vi "Simple Network Streams - Target.vi"() -> ()   [LabVIEW 2023]
doc: "Demonstrates how to use Network Streams to pass data and commands between two running VIs. This VI passes data to the host VI, based on the frequency specified by the host VI."
uses:
  support/Network Stream Command.ctl
  support/Network Stream Global Stop.vi
  <vilib>/ErrorRing/Error Ring.xnode
  <resource>/objmgr/ni.dex.rc
panel:
  out "Write Backlog":i32
  in  "Write Speed":u16(ring)=1 items=["Fast (10 ms)", "Slow (20 ms)"]
  out "Frequency":dbl(knob) scale=10.0..100.0
  in  "Stop":bool
  # "Overview: Demonstrates how to use Network Streams to pass data and commands between two running VIs.\nRequirements: Windows\nInstructions:\n1. Run this VI.\n2. Open Simple Network Streams - Host.vi and follow the instructions on its front panel."
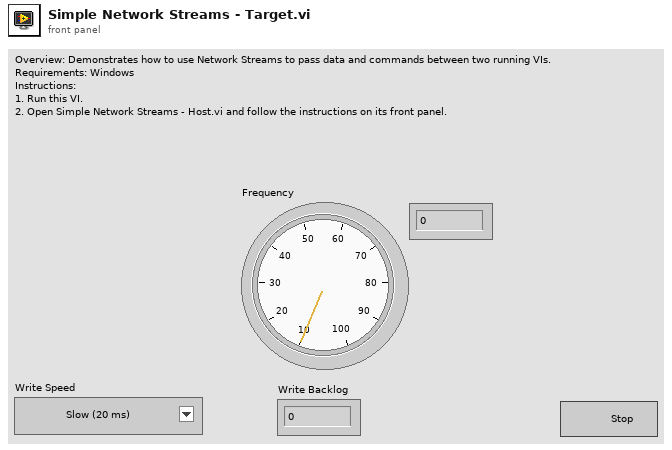
[diagram p1: front panel]
types:
  T1 = typedef "Network Stream Command.ctl" = cluster{"Message":string, "Message Data":variant}
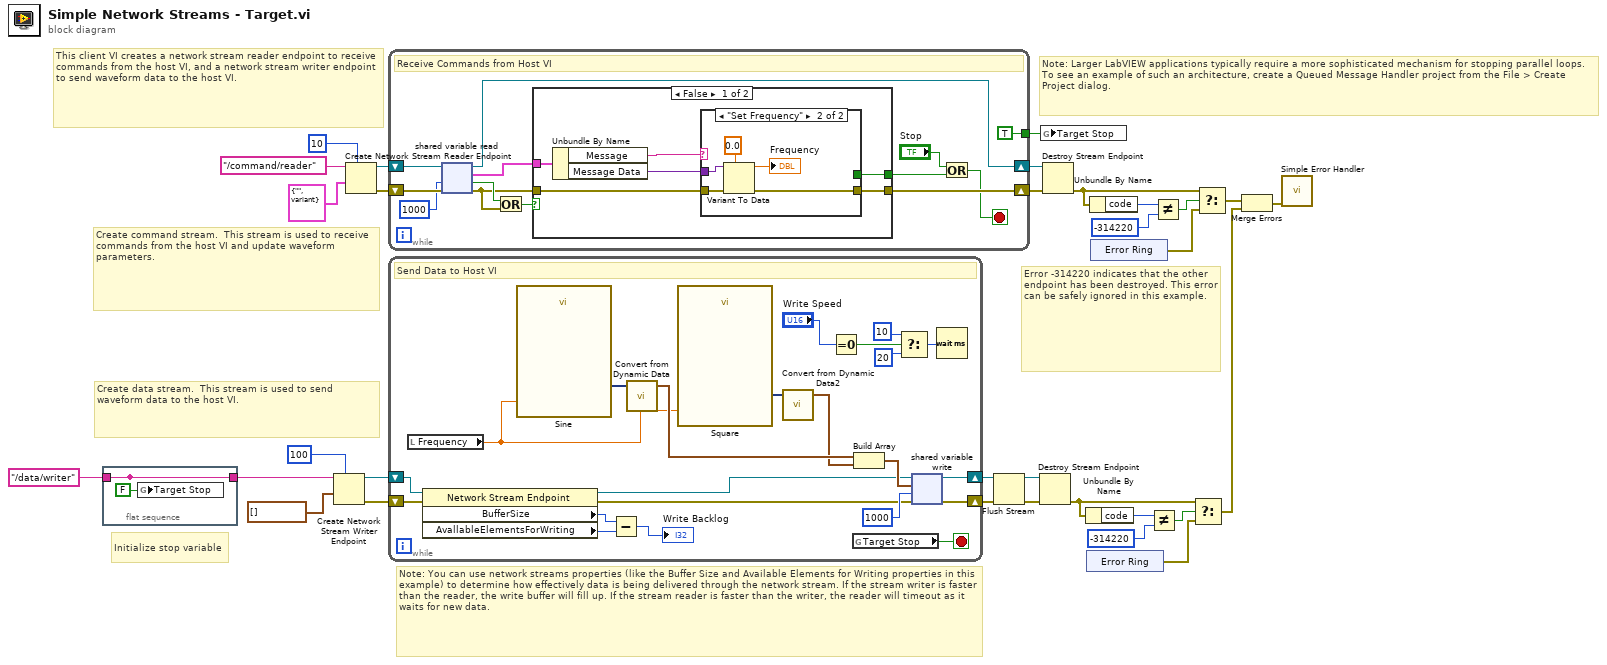
[diagram p0: block diagram]
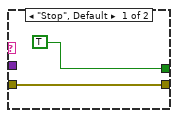
[diagram p2: hidden frame]
diagram:
  # "Initialize stop variable"
  # "This client VI creates a network stream reader endpoint to receive commands from the host VI, and a network stream writer endpoint to send waveform data to the host VI."
  # "Note: You can use network streams properties (like the Buffer Size and Available Elements for Writing properties in this example) to determine how effectively data is being delivered through the network stream. If the stream writer is faster than the reader, the write buffer will fill up. If the stream reader is faster than the writer, the reader will timeout as it waits for new data."
  # "Note: Larger LabVIEW applications typically require a more sophisticated mechanism for stopping parallel loops. To see an example of such an architecture, create a Queued Message Handler project from the File > Create Project dialog."
  # "Error -314220 indicates that the other endpoint has been destroyed. This error can be safely ignored in this example."
  # "Create command stream.  This stream is used to receive commands from the host VI and update waveform parameters."
  # "Create data stream.  This stream is used to send waveform data to the host VI."
  n1 = flat-sequence {
    tunnel: [w32] -> _
    tunnel: [w32] -> w1
    tunnel: "/data/writer" ("reader url") -> [w32]
    frame #0 {
      n2 = global write "Network Stream Global Stop.vi" "Target Stop"(FALSE ("Host Stop")) -> ()
    }
  }
  n3 = Create Network Stream Writer Endpoint(7:100 ("writer buffer size"), 9:waveform(dbl)[] [], 11:w1) -> (0:w31:errorcluster, 3:w30:refnum<k21>)  [unwired: 4 in]
  n4 = Create Network Stream Reader Endpoint(7:10 ("reader buffer size"), 9:T1 {"Message"="", "Message Data"=variant} ("Message Cluster"), 11:"/command/reader" ("reader url")) -> (0:w26:errorcluster, 3:w27:refnum<k21>)  [unwired: 4 in]
  n5 = while "Host->Target Command Reader" {
    shift-right: [w42] -> w25
    shift-left: w26 -> [w46]
    shift-right: [w44] -> w24
    shift-left: w27 -> [w45]
    tunnel: [TRUE] -> w3
    stop <- w38 stop-if-true
    # "Receive Commands from Host VI"
    n6 = shared-variable-read(w45, w46, 1000 ("timeout ms")) -> (w44:refnum<k21>, w35:errorcluster, w37:bool, w40:T1)
    n7 = Or(x=w37, y=w35) -> (x .or. y?=w36:bool)
    n8 = case shown="False" w36 {
      tunnel: w35 -> [w52 w60]
      tunnel: [w51 w60] -> w42
      tunnel: w40 -> [w49 _]
      tunnel: [w50 _] -> w39
      frame False {
        n9 = Unbundle By Name(w49) -> ("Message"=w48:string, "Message Data"=w47:variant)
        n10 = case shown="\"Set Frequency\"" w48 {
          tunnel: w52 -> [w54 w58]
          tunnel: [w54 w57] -> w51
          tunnel: w47 -> [_ w56]
          tunnel: [TRUE _] -> w50
          frame "Stop", Default {
          }
          frame "Set Frequency" {
            n11 = Variant To Data(error in=w58, type=0.0, Variant=w56) -> (data=→"Frequency":dbl, error out=w57:errorcluster)
          }
        }
      }
      frame True {
      }
    }
    n12 = Or(x="Stop", y=w39) -> (x .or. y?=w38:bool)
  }
  n13 = while "Target->Host Data Writer" {
    shift-right: [w63] -> w20
    shift-left: w31 -> [w65]
    shift-right: [w68] -> w29
    shift-left: w30 -> [w67]
    stop <- w61 stop-if-true
    # "Send Data to Host VI"
    n14 = local read "Frequency"() -> (w62:dbl)
    n15 = property class="Network Stream Endpoint"(reference=w67, error in=w65) -> (reference out=w66:refnum<k21>, error out=w64:errorcluster, "BufferSize"=w70:i32, "AvallableElementsForWriting"=w71:i32)
    n16 = call "Sine"("Frequency"=w62) -> ("Sine with Uniform Noise"=w81:dynamicdata)  [unwired: 13 in, 1 out]
    n17 = Subtract(x=w70, y=w71) -> (x-y=→"Write Backlog":i32)
    n18 = call "Convert from Dynamic Data"("Dynamic Data Type"=w81) -> ("Waveform"=w80:waveform(dbl))  [unwired: 3 in]
    n19 = call "Square"("Frequency"=w62) -> ("Square with Uniform Noise"=w77:dynamicdata)  [unwired: 13 in, 1 out]
    n20 = call "Convert from Dynamic Data2"("Dynamic Data Type"=w77) -> ("Waveform"=w79:waveform(dbl))  [unwired: 3 in]
    n21 = Equal To 0?(x="Write Speed") -> (x = 0?=w73:bool)
    n22 = global read "Network Stream Global Stop.vi" "Target Stop"() -> (w61:bool)
    n23 = Build Array(w80, w79) -> (w78:waveform(dbl)[])
    n24 = Select(t=u32 10 ("milliseconds to wait"), s=w73, f=u32 20 ("milliseconds to wait")) -> (s? t:f=w75:u32)
    n25 = shared-variable-write(w66, w64, w78, 1000 ("timeout ms")) -> (w68:refnum<k21>, w63:errorcluster)  [unwired: 1 out]
    n26 = Wait (ms)(milliseconds to wait=w75) -> ()  [unwired: 1 out]
  }
  n27 = Flush Stream(8:w20, 11:w29) -> (0:w19:errorcluster, 3:w21:refnum<k21>)  [unwired: 2 in, 1 out]
  n28 = Destroy Stream Endpoint(8:w19, 11:w21) -> (0:w5:errorcluster)
  n29 = global write "Network Stream Global Stop.vi" "Target Stop"(w3) -> ()
  n30 = Destroy Stream Endpoint(8:w25, 11:w24) -> (0:w11:errorcluster)
  n31 = Unbundle By Name(w5) -> ("code"=w9:i32)
  n32 = xnode "Error Ring"() -> ("error out"=w6:errorcluster)
  n33 = Unbundle By Name(w11) -> ("code"=w12:i32)
  n34 = xnode "Error Ring"() -> ("error out"=w15:errorcluster)
  n35 = Not Equal?(x=w9, y=-314220) -> (x != y?=w7:bool)
  n36 = Not Equal?(x=w12, y=-314220) -> (x != y?=w14:bool)
  n37 = Select(t=w5, s=w7, f=w6) -> (s? t:f=w4:errorcluster)
  n38 = Select(t=w11, s=w14, f=w15) -> (s? t:f=w10:errorcluster)
  n39 = Merge Errors(w10, w4) -> (w18:errorcluster)
  n40 = call <vilib>:"Simple Error Handler.vi"("error in (no error)"=w18) -> ()  [unwired: 4 in, 5 out]
